vi "FestoCPX.Valve(2out0in).vi"(4 "Delay [ms] (0)":u32, 8 "error in (no error)":errorcluster, 9 "Position":T2, 10 "Valve outputs":T1[](array[typedef])) -> (0 "error out":errorcluster)   [LabVIEW 2016]
uses:
  Station/Station.ValvePosition.ctl
  FestoCPX.DO.Signal.ctl
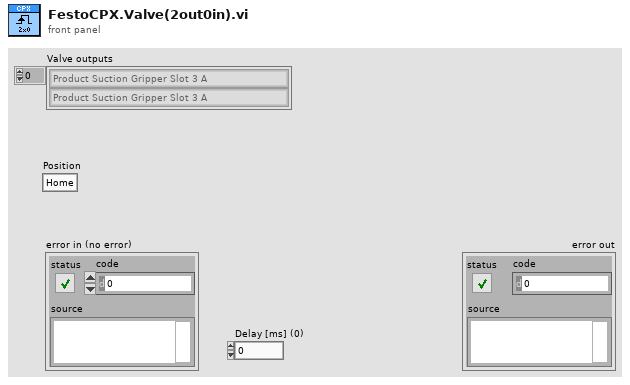
[diagram p1: front panel]
types:
  T1 = typedef "FestoCPX.DO.Signal.ctl" = enum16{"Safety Reset", "Air Main Valve", "Door Lock", "Button LED Start", "Button LED Stop", "Button LED Control", "Traffic LED Red", "Traffic LED Orange", "Traffic LED Green", "Horn", "Laser Interlock", "Laser Trigger", "Laser Fume Extractor", "Product Suction Gripper Slot 1 A", "Product Suction Gripper Slot 1 B", "Product Suction Gripper Slot 2 A", "Product Suction Gripper Slot 2 B", "Product Suction Gripper Slot 3 A", "Product Suction Gripper Slot 3 B", "Product Suction Gripper Slot 4 A", "Product Suction Gripper Slot 4 B", "Product Suction Gripper Final A", "Product Suction Gripper Final B", "Lamp", "Q1 Product Move Work", "Q1 Product Move Home", "Q2 Table Turn Work", "Q2 Table Turn Home", "Q3 Product Lift A", "Q3 Product Lift B", "Q4 Product Arm OK", "Q4 Product Arm NOK", "Q5 Product Arm Work", "Q6 Product BlowOut A", "Q6 Product BlowOut B"}
  T2 = typedef "Station.ValvePosition.ctl" = enum16{"Home", "Work"}
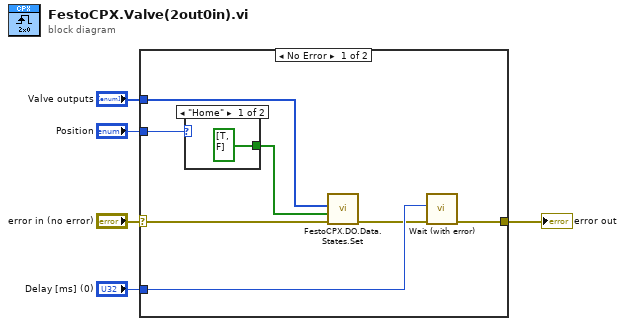
[diagram p0: block diagram]
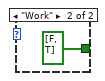
[diagram p2: hidden frame]
diagram:
  n1 = case shown="No Error" "error in (no error)" {
    selector: "error in (no error)" -> [w9 w15]
    tunnel: "Position" -> [w12 _]
    tunnel: [w10 w15] -> w4
    tunnel: "Delay [ms] (0)" -> [w11 _]
    tunnel: "Valve outputs" -> [w6 _]
    frame No Error {
      n2 = case shown="\"Home\"" w12 {
        tunnel: [bool[] [TRUE, FALSE] bool[] [FALSE, TRUE]] -> w7
        frame "Home" {
        }
        frame "Work" {
        }
      }
      n3 = call "FestoCPX.DO.Data.States.Set.vi"("error in (no error)"=w9, "State"=w7, "CPX.DO"=w6) -> ("error out"=w8:errorcluster)  [unwired: 8 in]
      n4 = call "Wait (with error).vi"("error in (no error)"=w8, "milliseconds to wait"=w11) -> ("error out"=w10:errorcluster)  [unwired: 8 in, 1 out]
    }
    frame Error {
    }
  }
  "error out" <- w4
